vi "Main.vi"() -> ()   [LabVIEW 2024]
uses:
  <vilib>/vision/Image Controls.llb/IMAQ Image.ctl
panel:
  out "Time":string
  out "Date":string
  in  "Upload the Scan":path
  in  "Stop":bool caption="Save"
  in  "Save":bool
  in  "Predict":bool caption="Inspect"
  out "Error":errorcluster
  out "Scan Image":T1(plugin-control)
  out "Possible Recovery time":dbl caption="month(s)"
  out "Possible Stroke type":string
  # "Real-Time Stroke Recovery Prediction Using MRI Imaging using \nLabVIEW-Python Integrated Approach"
  # "-Ajay Aruljothi\nBio-Tech Instrumentatoin Project"
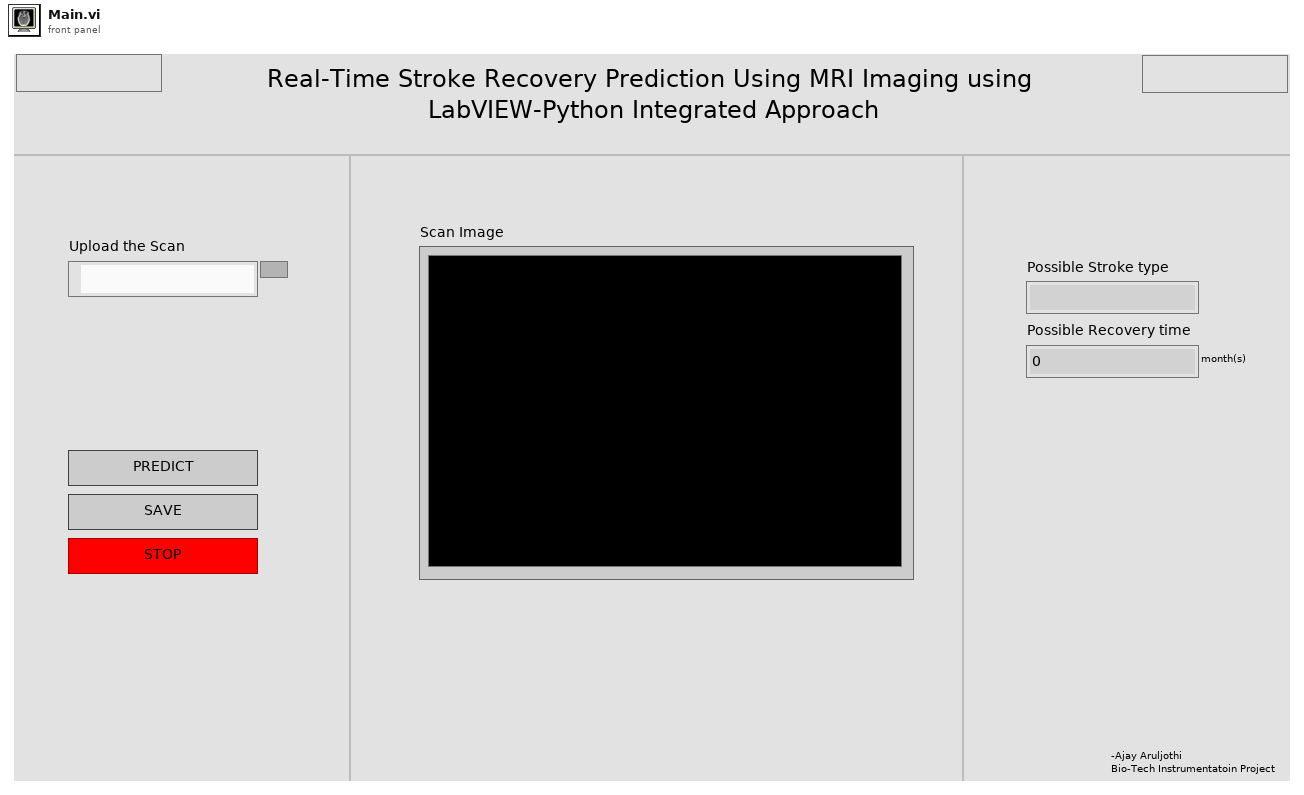
[diagram p1: front panel]
types:
  T1 = typedef "IMAQ Image.ctl" = refnum<image>
  T2 = cluster{"Upload the Scan":path, "Predict":bool, "Save":bool, "Stop":bool, "Main Case":string, "Scan Img":T1, "Stroke Type":string, "Pbl. rvy. ti.":dbl, "Temp. img. path":string, "Pre. LV. path":path, "Py. fun. name":string, "Py. Ref. in":refnum<k35>, "Py. Ref. out":refnum<k35>, "Error out":refnum<file>}
  T3 = cluster{"stroke_type":string, "recovery_months":dbl}
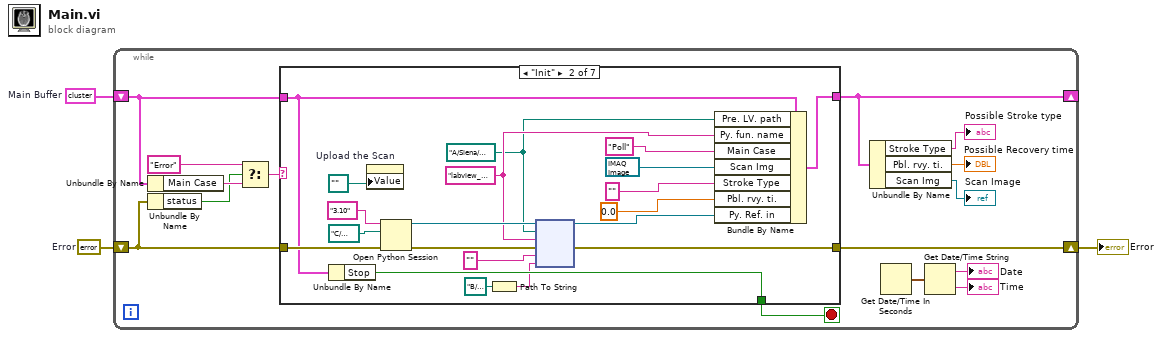
[diagram p0: block diagram]
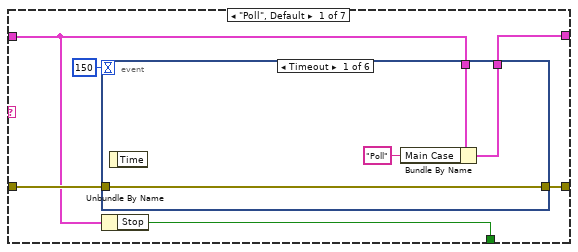
[diagram p2: hidden frame]
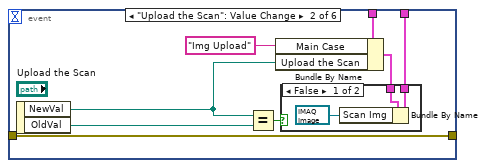
[diagram p3: hidden frame]
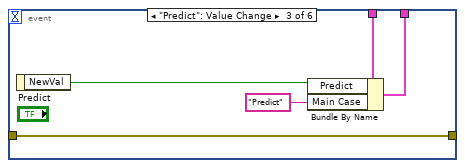
[diagram p5: hidden frame]
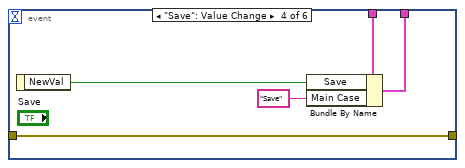
[diagram p6: hidden frame]
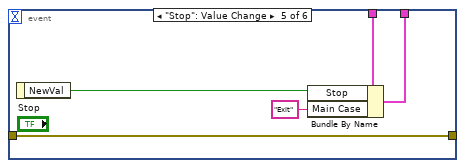
[diagram p7: hidden frame]
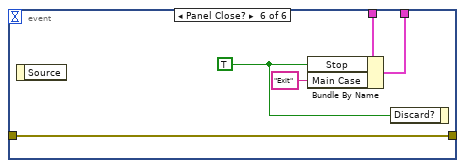
[diagram p8: hidden frame]
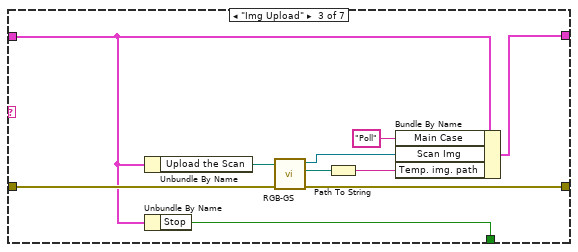
[diagram p9: hidden frame]
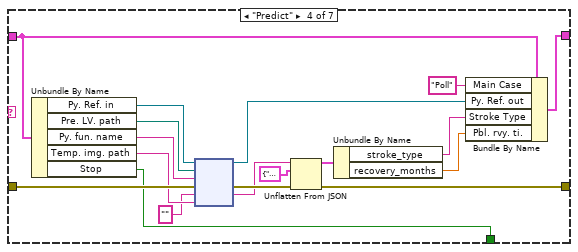
[diagram p10: hidden frame]
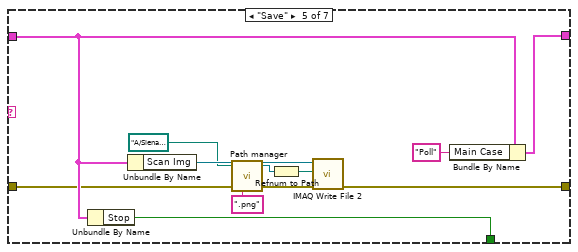
[diagram p11: hidden frame]
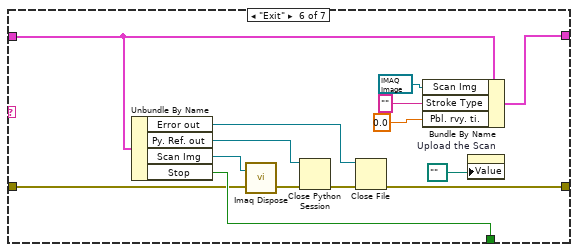
[diagram p12: hidden frame]
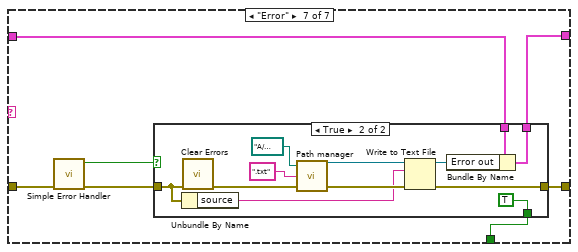
[diagram p13: hidden frame]
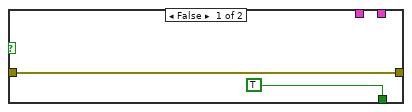
[diagram p14: hidden frame]
diagram:
  w2 = errorcluster {"status"=FALSE, "code"=0, "source"=""}  # Error
  w3 = T2 {"Upload the Scan"=path "", "Predict"=FALSE, "Save"=FALSE, "Stop"=FALSE, "Main Case"="Init", "Scan Img"=refnum, "Stroke Type"="", "Pbl. rvy. ti."=0.0, "Temp. img. path"="", "Pre. LV. path"=path "", "Py. fun. name"="", "Py. Ref. in"=refnum, "Py. Ref. out"=refnum, "Error out"=refnum}  # Main Buffer
  n1 = while {
    shift-right: [w11] -> _
    shift-left: w3 -> [w18]
    shift-right: [w16] -> w1
    shift-left: w2 -> [w15]
    stop <- w17 stop-if-true
    n2 = Unbundle By Name(w18) -> ("Main Case"=w13:string)
    n3 = Unbundle By Name(w15) -> ("status"=w7:bool)
    n4 = Select(t="Error", s=w7, f=w13) -> (s? t:f=w14:string)
    n5 = case shown="\"Init\"" w14 {
      tunnel: w18 -> [w20 w76 w84 w105 w117 w131 w136]
      tunnel: [w23 w78 w90 w107 w119 w130 w135] -> w11
      tunnel: [w19 w75 w83 w94 w118 w134 w137] -> w17
      tunnel: w15 -> [w22 w77 w87 w108 w114 w133 w141]
      tunnel: [w21 w68 w85 w93 w116 w122 w139] -> w16
      frame "Poll", Default {
        n6 = event shown="[0] Timeout" {
          selector: _ -> [_ _ _ _ _ _]
          dyn-events: _ -> [_ _ _ _ _ _]
          timeout: 150 -> [_ _ _ _ _ _]
          tunnel: w20 -> [w28 w36 w45 w50 w55 w60]
          tunnel: [w26 w30 w44 w49 w54 w59] -> w23
          tunnel: w22 -> [w25 w34 w41 w46 w51 w56]
          tunnel: [w25 w34 w41 w46 w51 w56] -> w21
          event Timeout {
            n7 = event-data() -> ()  [unwired: 1 in, 1 out]
            n8 = Bundle By Name(cluster=w28, "Main Case"="Poll") -> (w26:T2)
          }
          event "Upload the Scan": Value Change {
            n9 = event-data() -> ("NewVal"=w33:path, "OldVal"=w32:path)  [unwired: 1 in]
            n10 = Equal?(x=w33, y=w32) -> (x = y?=w31:bool)
            n11 = Bundle By Name(cluster=w36, "Main Case"="Img Upload" ("Case"), "Upload the Scan"=w33) -> (w29:T2)
            n12 = case shown="False" w31 {
              tunnel: [w38 w40] -> w30
              tunnel: w29 -> [w39 w40]
              frame False {
                n13 = Bundle By Name(cluster=w39, "Scan Img"=T1 refnum ("Result")) -> (w38:T2)
              }
              frame True {
              }
            }
          }
          event "Predict": Value Change {
            n14 = event-data() -> ("NewVal"=w43:bool)  [unwired: 1 in]
            n15 = Bundle By Name(cluster=w45, "Predict"=w43, "Main Case"="Predict") -> (w44:T2)
          }
          event "Save": Value Change {
            n16 = event-data() -> ("NewVal"=w48:bool)  [unwired: 1 in]
            n17 = Bundle By Name(cluster=w50, "Save"=w48, "Main Case"="Save") -> (w49:T2)
          }
          event "Stop": Value Change {
            n18 = event-data() -> ("NewVal"=w53:bool)  [unwired: 1 in]
            n19 = Bundle By Name(cluster=w55, "Stop"=w53, "Main Case"="Exit") -> (w54:T2)
          }
          event Panel Close? {
            w58 = TRUE ("Stop")
            n20 = event-data() -> ()  [unwired: 1 in, 1 out]
            n21 = Bundle By Name(cluster=w60, "Stop"=w58, "Main Case"="Exit") -> (w59:T2)
            n22 = event-data("Discard?"=w58) -> ()  [unwired: 1 in, 1 out]
          }
        }
        n23 = Unbundle By Name(w20) -> ("Stop"=w19:bool)
      }
      frame "Init" {
        w62 = "labview_predict_from_path" ("Py. fun. name")
        w61 = path "A:/Siena/Bio-Tech Instrumentation/Stroke recovery time perdiction/Py. Code/Stroke_Recovery_prediction_LabVIEW_Node.py" ("module path")
        n24 = Unbundle By Name(w76) -> ("Stop"=w75:bool)
        n25 = property on="Upload the Scan" class="Path"("Value"=path "" ("Upload the Scan")) -> ()  [unwired: 2 in, 2 out]
        n26 = Open Python Session(python version="3.10" ("Python version"), python path=path "C:/Users/ajaya/AppData/Local/Programs/Python/Python310/python.exe" ("Python path"), 3:w77) -> (session out=w67:refnum<k35>, error out=w69:errorcluster)
        n27 = Path To String(path=path "B:/sample/1.png") -> (string=w64:string)
        n28 = node(w67, w61, w62, w69, "", w64) -> (w66:refnum<k35>, w68:errorcluster)  [unwired: 2 in, 2 out]
        n29 = Bundle By Name(cluster=w76, "Pre. LV. path"=w61, "Py. fun. name"=w62, "Main Case"="Poll", "Scan Img"=T1 refnum, "Stroke Type"="", "Pbl. rvy. ti."=0.0, "Py. Ref. in"=w66) -> (w78:T2)
      }
      frame "Img Upload" {
        n30 = Unbundle By Name(w84) -> ("Upload the Scan"=w88:path)
        n31 = Unbundle By Name(w84) -> ("Stop"=w83:bool)
        n32 = call "RGB-GS.vi"("error in"=w87, "Upload the Scan"=w88) -> ("error out"=w85:errorcluster, "File Path"=w86:path, "Refnum out"=w81:T1)  [unwired: 7 in]
        n33 = Path To String(path=w86) -> (string=w82:string)
        n34 = Bundle By Name(cluster=w84, "Main Case"="Poll" ("Case"), "Scan Img"=w81, "Temp. img. path"=w82) -> (w90:T2)
      }
      frame "Predict" {
        n35 = Unbundle By Name(w105) -> ("Py. Ref. in"=w99:refnum<k35>, "Pre. LV. path"=w102:path, "Py. fun. name"=w100:string, "Temp. img. path"=w103:string, "Stop"=w94:bool)
        n36 = node ("Python Node")(w99, w102, w100, w108, "", w103) -> (w92:refnum<k35>, w97:errorcluster, w91:string)  [unwired: 1 in, 2 out]
        n37 = Unflatten From JSON(JSON string=w91, type and defaults=T3 {"stroke_type"="", "recovery_months"=0.0}, error in (no error)=w97) -> (value=w104:T3, error out=w93:errorcluster)  [unwired: 4 in]
        n38 = Unbundle By Name(w104) -> ("stroke_type"=w96:string, "recovery_months"=w95:dbl)
        n39 = Bundle By Name(cluster=w105, "Main Case"="Poll", "Py. Ref. out"=w92, "Stroke Type"=w96, "Pbl. rvy. ti."=w95) -> (w107:T2)
      }
      frame "Save" {
        n40 = Unbundle By Name(w117) -> ("Stop"=w118:bool)
        n41 = Unbundle By Name(w117) -> ("Scan Img"=w113:T1)
        n42 = call "Path manager.vi"("error in"=w114, "File Type"=".png", "File Path"=path "A:/Siena/Bio-Tech Instrumentation/Stroke recovery time perdiction/LabVIEW/Save image") -> ("error out"=w115:errorcluster, "refnum out"=w110:refnum<file>)  [unwired: 1 in]
        n43 = Refnum to Path(1:w110) -> (0:w109:path)
        n44 = call-poly "IMAQ Write File 2"("error in (no error)"=w115, "File Path"=w109, "Image"=w113) -> ("error out"=w116:errorcluster)  [unwired: 7 in, 1 out]
        n45 = Bundle By Name(cluster=w117, "Main Case"="Poll") -> (w119:T2)
      }
      frame "Exit" {
        n46 = Unbundle By Name(w131) -> ("Error out"=w121:refnum<file>, "Py. Ref. out"=w125:refnum<k35>, "Scan Img"=w132:T1, "Stop"=w134:bool)
        n47 = call "Imaq Dispose"("Image"=w132, "error in (no error)"=w133) -> ("error out"=w126:errorcluster)  [unwired: 4 in]
        n48 = Close Python Session(session in=w125, error in=w126) -> (11:w123:errorcluster)
        n49 = Close File(refnum=w121, error in=w123) -> (error out=w122:errorcluster)  [unwired: 1 out]
        n50 = Bundle By Name(cluster=w131, "Scan Img"=T1 refnum, "Stroke Type"="", "Pbl. rvy. ti."=0.0 ("Possible recovery time")) -> (w130:T2)
        n51 = property on="Upload the Scan" class="Path"("Value"=path "" ("Upload the Scan")) -> ()  [unwired: 2 in, 2 out]
      }
      frame "Error" {
        n52 = call <vilib>:"Simple Error Handler.vi"("error in (no error)"=w141) -> ("error?"=w138:bool, "error out"=w140:errorcluster)  [unwired: 4 in, 3 out]
        n53 = case shown="True" w138 {
          tunnel: w140 -> [w143 w147]
          tunnel: [w143 w153] -> w139
          tunnel: [TRUE TRUE] -> w137
          tunnel: w136 -> [w142 w150]
          tunnel: [w142 w148] -> w135
          frame False {
          }
          frame True {
            n54 = Unbundle By Name(w147) -> ("source"=w146:string)
            n55 = call <vilib>:"Clear Errors.vi"("error in (no error)"=w147) -> ("error out"=w145:errorcluster)  [unwired: 5 in, 1 out]
            n56 = call "Path manager.vi"("error in"=w145, "File Type"=".txt", "File Path"=path "A:/Siena/Bio-Tech Instrumentation/Stroke recovery time perdiction/LabVIEW/Error Log" ("file path (use dialog)")) -> ("error out"=w151:errorcluster, "refnum out"=w152:refnum<file>)  [unwired: 1 in]
            n57 = Write to Text File(file (use dialog)=w152, text=w146, error in=w151) -> (refnum out=w149:refnum<file>, error out=w153:errorcluster)  [unwired: 1 in, 1 out]
            n58 = Bundle By Name(cluster=w150, "Error out"=w149) -> (w148:T2)
          }
        }
      }
    }
    n59 = Unbundle By Name(w11) -> ("Stroke Type"=→"Possible Stroke type":string, "Pbl. rvy. ti."=→"Possible Recovery time":dbl, "Scan Img"=→"Scan Image":T1)
    n60 = Get Date/Time In Seconds() -> (seconds since 1Jan1904=w6:timestamp)
    n61 = Get Date/Time String(seconds (now)=w6) -> (date string=→"Date":string, time string=→"Time":string)  [unwired: 2 in]
  }
  "Error" <- w1
